vi "MU Mt Analyze Result Calculate Offset Error.vi"(8 "error in (no error)":errorcluster, 9 "MtTrackOffset":u8, 10 "Samples":u64, 11 "MtSync_AnalyzeResultHandle":T1) -> (0 "error out":errorcluster, 2 "MT_OffsetError":dbl[](array[numeric]), 3 "Return Value":u64)   [LabVIEW 2017, in "MU_3SL_interface.lvlib"]
uses:
  MU_3SL_interface.lvlib
  handles/mtSyncAnalyzeResultHandle.ctl
  lib/MU_3SL_interface.dll
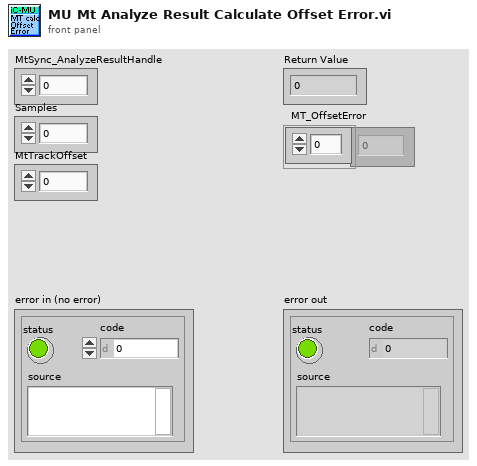
[diagram p1: front panel]
types:
  T1 = typedef "MU_3SL_interface.lvlib/mtSyncAnalyzeResultHandle.ctl" = u64
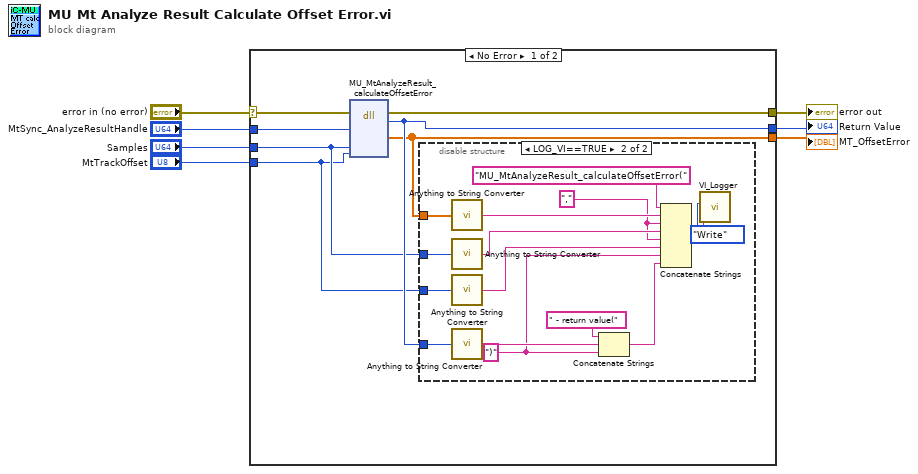
[diagram p0: block diagram]
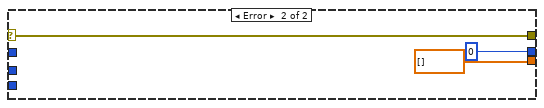
[diagram p3: hidden frame]
diagram:
  n1 = case shown="No Error" "error in (no error)" {
    selector: "error in (no error)" -> [w14 w32]
    tunnel: [w13 u64 0 ("Return Value")] -> w1
    tunnel: [w12 w32] -> w7
    tunnel: "MtSync_AnalyzeResultHandle" -> [w11 _]
    tunnel: "Samples" -> [w9 _]
    tunnel: [w10 dbl[] [] ("MT_OffsetError")] -> w3
    tunnel: "MtTrackOffset" -> [w8 _]
    frame No Error {
      n2 = dll-call lib="C:/Users/bes/AppData/Roaming/work/mu_9so/icsubmodules/soft_mu_3sl_master/lv_interface/lib/MU_3SL_interface**.*" fn="MU_MtAnalyzeResult_calculateOffsetError"(error in=w14, "analyzeResultHandle"=w11, "Samples"=w9, "MtTrackOffset"=w8) -> (error out=w12:errorcluster, "Return Value"=w13:u64, "MT_OffsetError"=w10:dbl[])  [unwired: 6 in, 1 out]
      n3 = disable-structure shown="LOG_VI==TRUE" {
        disable-tunnel: w13 -> [_ w25]
        disable-tunnel: w10 -> [_ w22]
        disable-tunnel: w9 -> [_ w19]
        disable-tunnel: w8 -> [_ w18]
        frame condition #0 {
        }
        frame condition #1 (active) {
          w20 = "," ("string")
          w16 = ")" ("string")
          n4 = call "Anything to String Converter.vi"("anything"=w22) -> ("String"=w23:string)
          n5 = call "Anything to String Converter.vi"("anything"=w19) -> ("String"=w21:string)
          n6 = call "Anything to String Converter.vi"("anything"=w18) -> ("String"=w17:string)
          n7 = call "Anything to String Converter.vi"("anything"=w25) -> ("String"=w24:string)
          n8 = Concatenate Strings(" - return value(" ("string"), w24, w16) -> (w15:string)
          n9 = Concatenate Strings("MU_MtAnalyzeResult_calculateOffsetError(" ("Info in"), w23, w20, w21, w20, w17, w16, w15) -> (w27:string)
          n10 = call "VI_Logger.vi"("Action (Read)"=enum16{"Write", "Read"}."Write", "Info in"=w27) -> ()  [unwired: 8 in, 2 out]
        }
      }
    }
    frame Error {
    }
  }
  "error out" <- w7
  "MT_OffsetError" <- w3
  "Return Value" <- w1
